vi "....SPEECH RECOGNITION only...vi"() -> ()   [LabVIEW 2018]
panel:
  in  "CMD List":string[](array[string])
  in  "Error In":errorcluster
  out "Error Out":errorcluster
  in  "Exit":bool
  out "Voice Command":string
  # "Speech Recognition System"
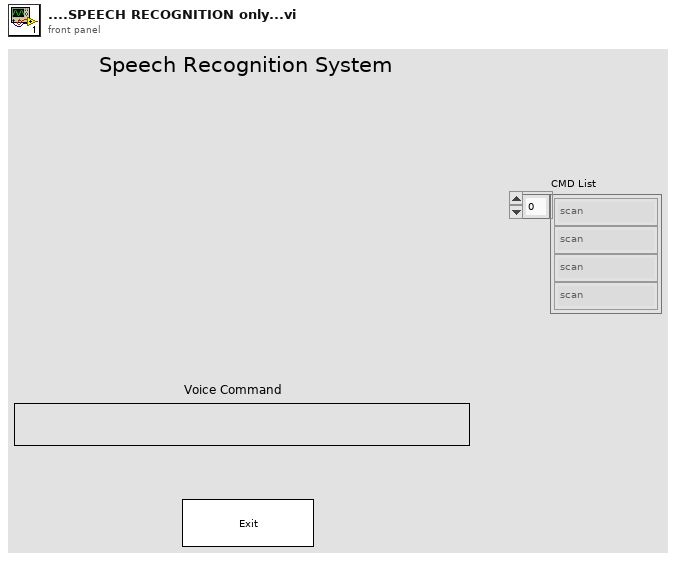
[diagram p1: front panel]
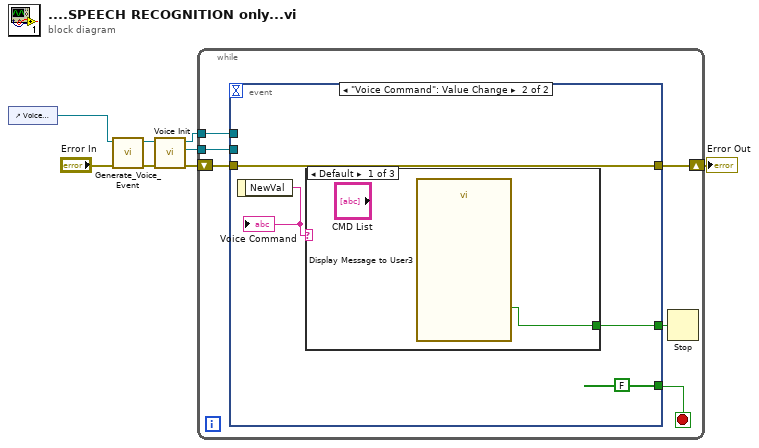
[diagram p0: block diagram]
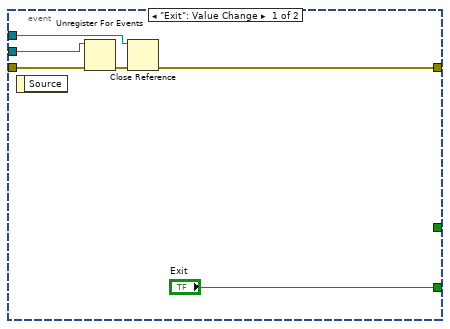
[diagram p2: hidden frame]
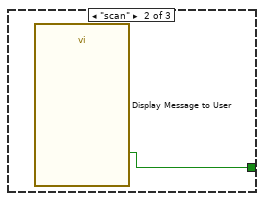
[diagram p3: hidden frame]
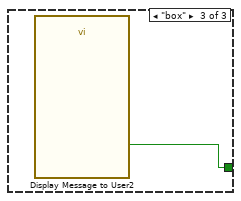
[diagram p4: hidden frame]
diagram:
  n1 = control-ref of="Voice Command"() -> (w7:refnum<vi>)
  n2 = call "Generate_Voice_Event.vi"("Error In"="Error In", "String in"=w7) -> ("Error Out"=w6:errorcluster, "String out"=w8:refnum<vi>)  [unwired: 8 in]
  n3 = call "Voice Init.vi"("Error In"=w6, "Text"=w8) -> ("Error Out"=w4:errorcluster, "Event Callback"=w1:refnum<k27>, "Reference"=w5:refnum<k24>)  [unwired: 7 in]
  n4 = while {
    tunnel: w5 -> [w13]
    shift-right: [w11] -> w3
    shift-left: w4 -> [w12]
    tunnel: w1 -> [w10]
    stop <- w14 stop-if-true
    n5 = event shown="[1] \"Voice Command\": Value Change" {
      selector: _ -> [_ _]
      dyn-events: _ -> [_ _]
      timeout: _ -> [_ _]
      tunnel: ["Exit" FALSE ("Exit")] -> w14
      tunnel: w13 -> [w19 _]
      tunnel: w12 -> [w17 w24]
      tunnel: [w16 w24] -> w11
      tunnel: w10 -> [w15 _]
      tunnel: [_ w21] -> w9
      event "Exit": Value Change {
        n6 = event-data() -> ()  [unwired: 1 in, 1 out]
        n7 = Unregister For Events(event registration refnum=w15, error in=w17) -> (error out=w18:errorcluster)
        n8 = Close Reference(reference=w19, error in (no error)=w18) -> (error out=w16:errorcluster)
      }
      event "Voice Command": Value Change {
        n9 = event-data() -> ("NewVal"=w22:string)  [unwired: 1 in]
        "Voice Command" <- w22
        n10 = case shown="Default" w22 {
          tunnel: [w25 w26 w27] -> w21
          frame Default {
            n11 = call "Display Message to User3"() -> ("OK"=w25:bool)  [unwired: 10 in, 1 out]
          }
          frame "scan" {
            n12 = call "Display Message to User"() -> ("OK"=w26:bool)  [unwired: 10 in, 1 out]
          }
          frame "box" {
            n13 = call "Display Message to User2"() -> ("OK"=w27:bool)  [unwired: 10 in, 1 out]
          }
        }
      }
    }
    n14 = Stop(stop? (T)=w9) -> ()
  }
  "Error Out" <- w3
